vi "ReadoutTemp.vi"(2 "error in (no error)":errorcluster) -> (0 "error out":errorcluster, 1 "Temperature":dbl format="%#_8g")   [LabVIEW 2010]
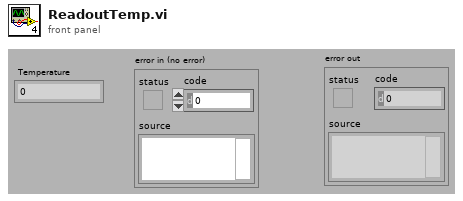
[diagram p1: front panel]
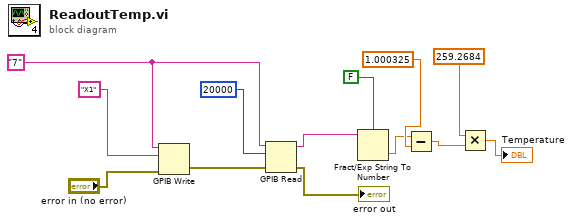
[diagram p0: block diagram]
diagram:
  w12 = "7"
  n1 = GPIB Write(0:w12, 1:"X1", 3:"error in (no error)") -> (6:w11:errorcluster)  [unwired: 2 in, 1 out]
  n2 = GPIB Read(0:w12, 1:20000, 3:w11) -> (5:w2:string, 7:→"error out":errorcluster)  [unwired: 2 in, 1 out]
  n3 = Fract/Exp String To Number(use system decimal point (T)=FALSE, string=w2) -> (number=w1:dbl)  [unwired: 2 in, 1 out]
  n4 = Subtract(x=w1, y=1.000325) -> (x-y=w7:dbl)
  n5 = Multiply(x=259.2684, y=w7) -> (x*y=→"Temperature":dbl)
